vi "Motic Get Frequency Index.vi"(8 "error in (no error)":errorcluster, 11 "camera":i32) -> (0 "error out":errorcluster, 2 "frequency index":i32, 3 "camera out":i32)   [LabVIEW 2012, in "MoticApi.lvlib"]
doc: "MOTICAPI int Motic_GetFrequencyIndex(MUCam_Handle camera);"
uses:
  MoticApi.lvlib
  MoticApi.dll
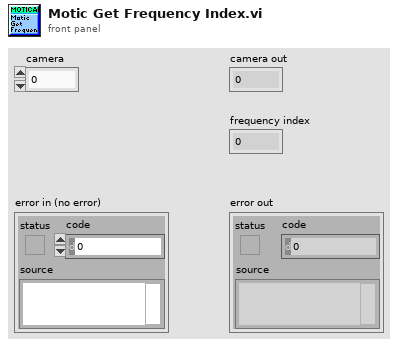
[diagram p1: front panel]
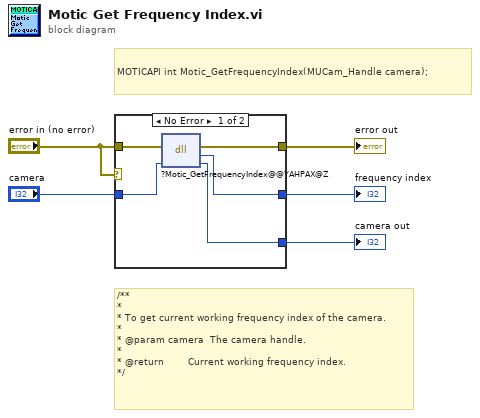
[diagram p0: block diagram]
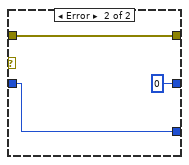
[diagram p2: hidden frame]
diagram:
  # "/**\n*\n* To get current working frequency index of the camera.\n*\n* @param camera  The camera handle.\n*\n* @return        Current working frequency index.\n*/"
  # "MOTICAPI int Motic_GetFrequencyIndex(MUCam_Handle camera);"
  n1 = case shown="No Error" "error in (no error)" {
    tunnel: [w10 0] -> w5
    tunnel: "camera" -> [w9 w12]
    tunnel: [w8 w12] -> w3
    tunnel: "error in (no error)" -> [w7 w13]
    tunnel: [w6 w13] -> w2
    frame No Error {
      n2 = dll-call lib="C:/Users/TTS-Digital/Desktop/MoticApi/MoticApi_git/MoticApi/MoticApi.*" fn="?Motic_GetFrequencyIndex@@YAHPAX@Z"(error in=w7, "camera"=w9) -> (error out=w6:errorcluster, w10:i32, "camera"=w8:i32)  [unwired: 2 in, 1 out]
    }
    frame Error {
    }
  }
  "frequency index" <- w5
  "camera out" <- w3
  "error out" <- w2
